vi "Generator.Generate Waveforms.vi"(6 "reset phase?":bool, 8 "error in (no error)":errorcluster, 11 "Instrument.DAQ":refnum<class "Instrument.DAQ.lvclass">) -> (0 "error out":errorcluster, 3 "Instrument.DAQ":refnum<class "Instrument.DAQ.lvclass">, 4 "phase reset":bool)   [LabVIEW 2019, in "Instrument.Lockin.lvlib" / "Instrument.DAQ.lvclass"]
uses:
  Instrument.DAQ.lvclass
  Instrument.DAQ.lvclass/Instrument.DAQ.ctl
  Typedefs/Status--enum.ctl
  5cf1a71e-08f9-4660-bbfa-1cc7de35ba4a.vi
  Generator/Generator.lvclass
  DAQmx/DAQmx.lvclass
panel:
  out "changed or first call?":bool
  out "reset":bool
  out "Min Queue Filled":bool
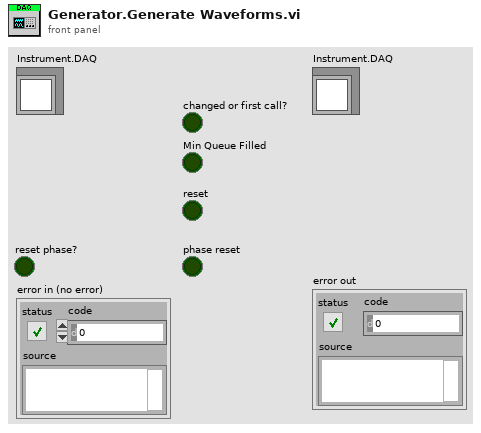
[diagram p1: front panel]
types:
  T1 = typedef "Instrument.Lockin.lvlib/Instrument.DAQ.lvclass/Status--enum.ctl" = enum16{"idle", "created", "started", "stopped", "sweeping"}
  T2 = typedef "Instrument.Lockin.lvlib/Instrument.DAQ.lvclass/DAQ.Sampling.Sampling--Cluster.ctl" = cluster{"Fs":dbl, "#s":i32}
  T3 = typedef "Generator.lvclass/AO.Channel--Cluster--Array.ctl" = T4[]
  T4 = typedef "Generator.lvclass/AO.Channel--Cluster.ctl" = cluster{"Enable?":bool, "Channel":i32, "Amplitude":dbl, "Offset":dbl, "Frequency":dbl, "Phase":dbl, "Function":T5, "Sweeping?":bool, "Limit AC?":bool, "Limit DC?":bool, "Duty Cycle?":bool, "Duty Cycle":dbl}
  T5 = typedef "Generator.lvclass/AO.Channel.Function--Enum.ctl" = enum16{"sine", "square", "triangle", "saw"}
  T6 = typedef "Instrument.Lockin.lvlib/Instrument.DAQ.lvclass/REF.Channel--Cluster--Array.ctl" = T7[]
  T7 = typedef "Instrument.Lockin.lvlib/Instrument.DAQ.lvclass/REF.Channel--Cluster.ctl" = cluster{"Enable?":bool, "Channel":i32, "Frequency":dbl, "Phase":dbl, "TC":dbl, "Roll-Off":i32}
  T8 = typedef "Instrument.Lockin.lvlib/Instrument.DAQ.lvclass/Sweep.Configuration--Cluster.ctl" = cluster{"Sweep Time (s)":dbl, "Initial Wait (s)":dbl, "Return to Start":bool, "Channels":T9}
  T9 = typedef "Instrument.Lockin.lvlib/Instrument.DAQ.lvclass/Sweep.Channel--Cluster--Array.ctl" = T10[]
  T10 = typedef "Instrument.Lockin.lvlib/Instrument.DAQ.lvclass/Sweep.Channel--Cluster.ctl" = cluster{"Enable?":bool, "Channel":u16, "Start":dbl, "End":dbl, "Pattern":T11, "Table":dbl[]}
  T11 = typedef "Instrument.Lockin.lvlib/Instrument.DAQ.lvclass/Sweep.Pattern--Enum.ctl" = enum16{"Ramp /", "Ramp /\\", "Smooth Ramp _/", "Smooth Ramp _/\\_", "Table"}
  T12 = typedef "Generator.lvclass/Waveforms--Cluster.ctl" = cluster{"AO":waveform(dbl)[], "REF_X":waveform(dbl)[], "REF_Y":waveform(dbl)[]}
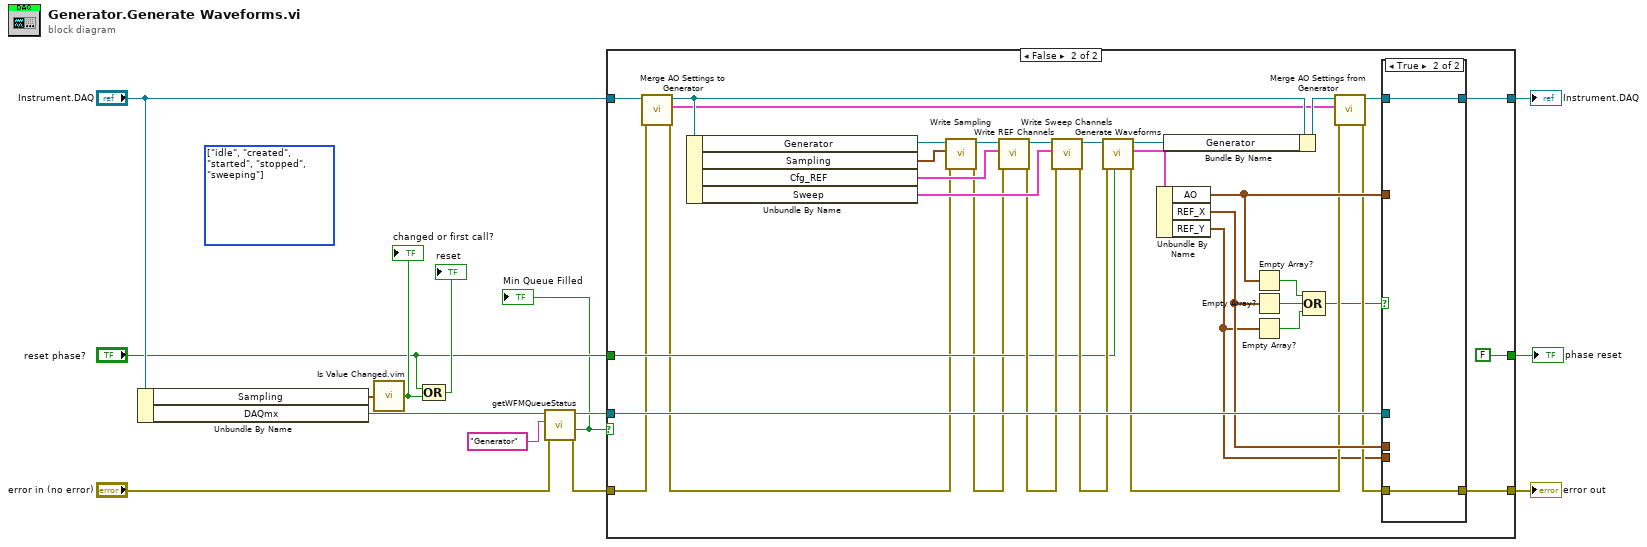
[diagram p0: block diagram]
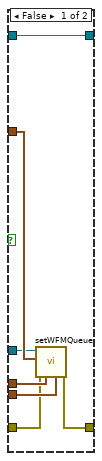
[diagram p3: hidden frame]
diagram:
  (unwired) T1[] [enum."idle", enum."created", enum."started", enum."stopped", enum."sweeping"] items=["idle", "created", "started", "stopped", "sweeping"] ("state")
  n1 = Unbundle By Name("Instrument.DAQ") -> ("Sampling"=w9:T2, "DAQmx"=w5:refnum<class "DAQmx.lvclass">)
  n2 = call "Is Value Changed.vim"("value"=w9) -> ("changed or first call?"=w8:bool)
  "changed or first call?" <- w8
  n3 = Compound Arithmetic op=OR("reset phase?", w8) -> (→"reset":bool)
  n4 = call "getWFMQueueStatus.vi"("error in (no error)"="error in (no error)", "instance"="Generator", "DAQmx in"=w5) -> ("error out"=w2:errorcluster, "Min AO Queue Filled"=w1:bool, "DAQmx out"=w10:refnum<class "DAQmx.lvclass">)  [unwired: 5 in, 1 out]
  "Min Queue Filled" <- w1
  n5 = case shown="False" w1 {
    tunnel: [w16 w19] -> w14
    tunnel: "reset phase?" -> [w15 w34]
    tunnel: w2 -> [w16 w24]
    tunnel: "Instrument.DAQ" -> [w17 w32]
    tunnel: [w17 w40] -> w13
    tunnel: w10 -> [_ w50]
    tunnel: [w15 FALSE] -> w11
    frame True {
    }
    frame False {
      n6 = call "Merge AO Settings to Generator.vi"("error in (no error)"=w24, "Instrument.DAQ in"=w32) -> ("error out"=w25:errorcluster, "AO Channels"=w18:T3, "Instrument.DAQ out"=w26:refnum<class "Instrument.DAQ.lvclass">)  [unwired: 7 in]
      n7 = Unbundle By Name(w26) -> ("Generator"=w44:refnum<class "Generator.lvclass">, "Sampling"=w45:T2, "Cfg_REF"=w47:T6, "Sweep"=w46:T8)
      n8 = call "Write Sampling.vi"("error in (no error)"=w25, "Sampling"=w45, "Generator in"=w44) -> ("error out"=w27:errorcluster, "Generator out"=w23:refnum<class "Generator.lvclass">)  [unwired: 7 in]
      n9 = call "Write REF Channels.vi"("error in (no error)"=w27, "REF Channels"=w47, "Generator in"=w23) -> ("error out"=w42:errorcluster, "Generator out"=w49:refnum<class "Generator.lvclass">)  [unwired: 7 in]
      n10 = call "Write Sweep Channels.vi"("error in (no error)"=w42, "Sweep Channels"=w46, "Generator in"=w49) -> ("error out"=w43:errorcluster, "Generator out"=w48:refnum<class "Generator.lvclass">)  [unwired: 7 in]
      n11 = call "Generate Waveforms.vi"("reset phase"=w34, "error in (no error)"=w43, "Generator.lvclass"=w48) -> ("error out"=w29:errorcluster, "Waveforms out"=w41:T12, "Generator.lvclass"=w39:refnum<class "Generator.lvclass">)  [unwired: 4 in, 2 out]
      n12 = Unbundle By Name(w41) -> ("AO"=w35:waveform(dbl)[], "REF_X"=w38:waveform(dbl)[], "REF_Y"=w22:waveform(dbl)[])
      n13 = Bundle By Name(cluster=w26, "Generator"=w39) -> (w31:refnum<class "Instrument.DAQ.lvclass">)
      n14 = Empty Array?(array=w35) -> (empty?=w21:bool)
      n15 = Empty Array?(array=w38) -> (empty?=w37:bool)
      n16 = Empty Array?(array=w22) -> (empty?=w36:bool)
      n17 = Compound Arithmetic op=OR(w21, w37, w36) -> (w20:bool)
      n18 = call "Merge AO Settings from Generator.vi"("error in (no error)"=w29, "configuration.AO Channels"=w18, "Instrument.DAQ in"=w31) -> ("error out"=w28:errorcluster, "Instrument.DAQ out"=w30:refnum<class "Instrument.DAQ.lvclass">)  [unwired: 7 in]
      n19 = case shown="True" w20 {
        tunnel: w50 -> [w55 _]
        tunnel: [w52 w59] -> w19
        tunnel: [w56 w58] -> w40
        tunnel: w28 -> [w51 w59]
        tunnel: w35 -> [w57 _]
        tunnel: w22 -> [w53 _]
        tunnel: w38 -> [w54 _]
        tunnel: w30 -> [w56 w58]
        frame False {
          n20 = call "setWFMQueue.vi"("REF_Y"=w53, "REF_X"=w54, "error in (no error)"=w51, "AO"=w57, "DAQmx in"=w55) -> ("error out"=w52:errorcluster)  [unwired: 5 in, 1 out]
        }
        frame True {
        }
      }
    }
  }
  "error out" <- w14
  "Instrument.DAQ" <- w13
  "phase reset" <- w11
